vi "Read Resource Config.vi"(8 "error in (no error)":errorcluster, 11 "Robot.lvclass":refnum<class "Robot.lvclass">) -> (0 "error out":errorcluster, 3 "Robot.lvclass":refnum<class "Robot.lvclass">)   [LabVIEW 2018, in "Robot.lvlib" / "Robot.lvclass"]
uses:
  Robot.lvclass
  Robot.lvclass/Robot.ctl
  PPLs/Configuration/Configuration.lvlibp/Configuration.lvclass
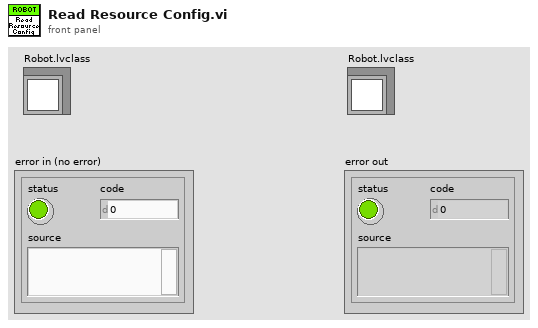
[diagram p1: front panel]
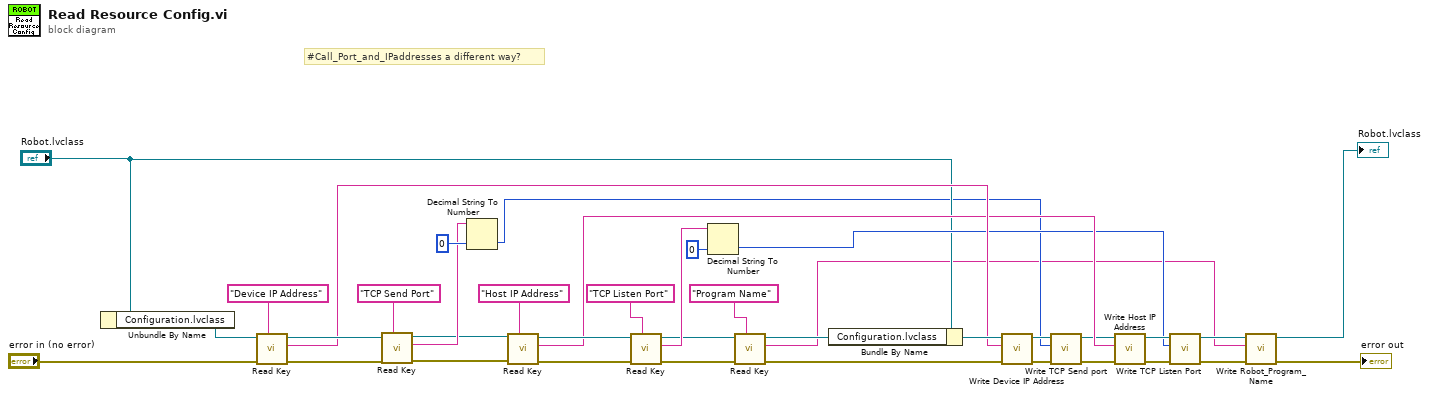
[diagram p0: block diagram]
diagram:
  # "#Call_Port_and_IPaddresses a different way?"
  n1 = Unbundle By Name("Robot.lvclass") -> ("Configuration.lvclass"=w23:refnum<class "Configuration.lvclass">)
  n2 = call "Read Key.vi"("Key:"="Device IP Address", "error in"="error in (no error)", "Configuration in"=w23) -> ("error out"=w26:errorcluster, "Value"=w21:string, "Configuration out"=w32:refnum<class "Configuration.lvclass">)  [unwired: 6 in]
  n3 = call "Read Key.vi"("Key:"="TCP Send Port", "error in"=w26, "Configuration in"=w32) -> ("error out"=w27:errorcluster, "Value"=w35:string, "Configuration out"=w33:refnum<class "Configuration.lvclass">)  [unwired: 6 in]
  n4 = Decimal String To Number(string=w35, default (0L)=u16 0 ("Remote port")) -> (number=w11:u16)  [unwired: 1 in, 1 out]
  n5 = call "Read Key.vi"("Key:"="Host IP Address", "error in"=w27, "Configuration in"=w33) -> ("error out"=w28:errorcluster, "Value"=w20:string, "Configuration out"=w34:refnum<class "Configuration.lvclass">)  [unwired: 6 in]
  n6 = call "Read Key.vi"("Key:"="TCP Listen Port", "error in"=w28, "Configuration in"=w34) -> ("error out"=w4:errorcluster, "Value"=w38:string, "Configuration out"=w5:refnum<class "Configuration.lvclass">)  [unwired: 6 in]
  n7 = Decimal String To Number(string=w38, default (0L)=u16 0 ("Read Port")) -> (number=w17:u16)  [unwired: 1 in, 1 out]
  n8 = call "Read Key.vi"("Key:"="Program Name", "error in"=w4, "Configuration in"=w5) -> ("error out"=w2:errorcluster, "Value"=w1:string, "Configuration out"=w3:refnum<class "Configuration.lvclass">)  [unwired: 6 in]
  n9 = Bundle By Name(cluster="Robot.lvclass", "Configuration.lvclass"=w3) -> (w22:refnum<class "Robot.lvclass">)
  n10 = call "Write Device IP Address.vi"("error in (no error)"=w2, "Device IP Address"=w21, "Robot in"=w22) -> ("error out"=w15:errorcluster, "Robot out"=w12:refnum<class "Robot.lvclass">)  [unwired: 7 in]
  n11 = call "Write TCP Send port.vi"("error in (no error)"=w15, "TCP Send port"=w11, "Robot in"=w12) -> ("error out"=w14:errorcluster, "Robot out"=w13:refnum<class "Robot.lvclass">)  [unwired: 7 in]
  n12 = call "Write Host IP Address.vi"("error in (no error)"=w14, "Host IP Address"=w20, "Robot in"=w13) -> ("error out"=w18:errorcluster, "Robot out"=w19:refnum<class "Robot.lvclass">)  [unwired: 7 in]
  n13 = call "Write TCP Listen Port.vi"("error in (no error)"=w18, "TCP Listen Port"=w17, "Robot in"=w19) -> ("error out"=w9:errorcluster, "Robot out"=w10:refnum<class "Robot.lvclass">)  [unwired: 7 in]
  n14 = call "Write Robot_Program_Name.vi"("error in (no error)"=w9, "Robot_Program_Name"=w1, "Robot in"=w10) -> ("error out"=→"error out":errorcluster, "Robot out"=→"Robot.lvclass":refnum<class "Robot.lvclass">)  [unwired: 7 in]
